vi "Remove Element.vi"(7 "Endpoint element key":string, 8 "error in (no error)":errorcluster, 10 "Token element":T1, 11 "OAuthAccessToken in":refnum<class "OAuthAccessToken.lvclass">) -> (0 "error out":errorcluster, 2 "Key":string, 3 "OAuthAccessToken out":refnum<class "OAuthAccessToken.lvclass">)   [LabVIEW 2013, in "OAuthAccessToken.lvclass"]
uses:
  OAuthAccessToken.lvclass
  OAuth2 Token Element -- enum.ctl
  OAuthAccessToken.lvclass/OAuthAccessToken.ctl
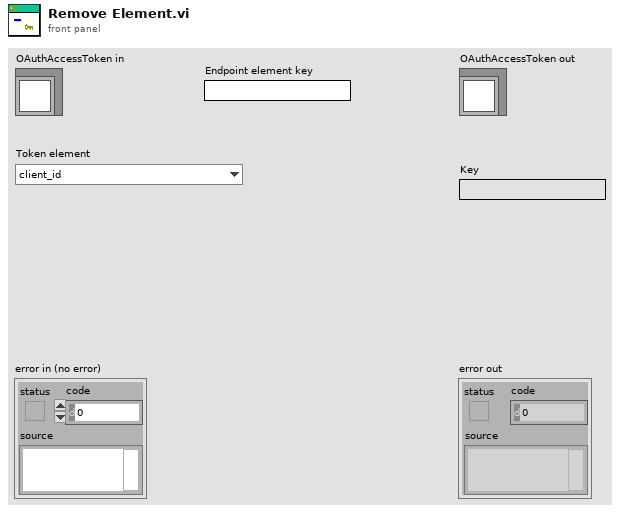
[diagram p1: front panel]
types:
  T1 = typedef "OAuthAccessToken.lvclass/OAuth2 Token Element -- enum.ctl" = enum16{"client_id", "client_secret", "response_type", "scope", "redirect_uri", "error", "error_description", "error_uri", "grant_type", "code", "access_token", "token_type", "expires_in", "username", "password", "refresh_token", "code_challenge", "code_verifier", "code_challenge_method", "endpoint element"}
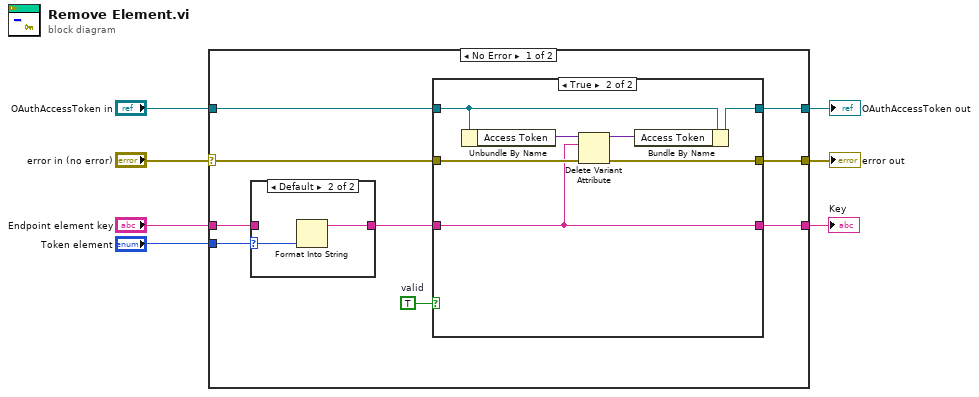
[diagram p0: block diagram]
diagram:
  n1 = case shown="No Error" "error in (no error)" {
    selector: "error in (no error)" -> [w12 w31]
    tunnel: [w11 w31] -> w6
    tunnel: [w15 w30] -> w4
    tunnel: "OAuthAccessToken in" -> [w16 w30]
    tunnel: "Token element" -> [w10 _]
    tunnel: "Endpoint element key" -> [w9 _]
    tunnel: [w8 _] -> w1
    frame No Error {
      w13 = TRUE  # valid
      n2 = case shown="Default" w10 {
        selector: w10 -> [_ w18]
        tunnel: [w17 w19] -> w14
        tunnel: w9 -> [w17 _]
        frame "endpoint element" {
        }
        frame Default {
          n3 = Format Into String(w18) -> (resulting string=w19:string)  [unwired: 3 in, 1 out]
        }
      }
      n4 = case shown="True" w13 {
        tunnel: w16 -> [w22 w29]
        tunnel: [w22 w28] -> w15
        tunnel: w14 -> [w20 w23]
        tunnel: w12 -> [w21 w26]
        tunnel: [w21 w25] -> w11
        tunnel: [w20 w23] -> w8
        frame False {
        }
        frame True {
          n5 = Unbundle By Name(w29) -> ("Access Token"=w24:variant)
          n6 = Delete Variant Attribute(4:w26, 6:w23, 7:w24) -> (0:w25:errorcluster, 3:w27:variant)  [unwired: 1 out]
          n7 = Bundle By Name(cluster=w29, "Access Token"=w27) -> (w28:refnum<class "OAuthAccessToken.lvclass">)
        }
      }
    }
    frame Error {
    }
  }
  "error out" <- w6
  "OAuthAccessToken out" <- w4
  "Key" <- w1
